vi "Atto DRY Interface upload Temperature Calibration Curve.vi"(8 "error in (no error)":errorcluster, 10 "Path":string, 11 "UserCurveNumber":u8) -> (0 "error out":errorcluster, 2 "Path out":string, 3 "function return":i32)   [LabVIEW 2016, in "attoDRYLib.lvlib"]
doc: "int32_t __cdecl AttoDRY_Interface_uploadTemperatureCalibrationCurve(\n uint8_t UserCurveNumber, char Path[]);"
uses:
  <userlib>/attoDRYLib/attoDRYLib.lvlib
  <userlib>/attoDRYLib/attoDRYLib.dll
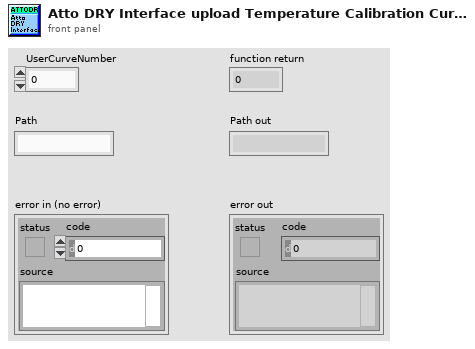
[diagram p1: front panel]
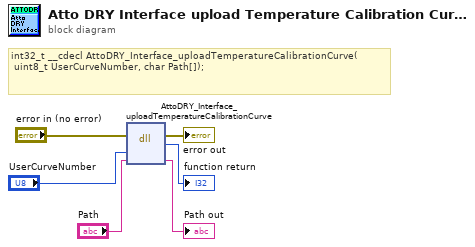
[diagram p0: block diagram]
diagram:
  # "int32_t __cdecl AttoDRY_Interface_uploadTemperatureCalibrationCurve(\n\tuint8_t UserCurveNumber, char Path[]);"
  n1 = dll-call lib="C:/Program Files (x86)/National Instruments/LabVIEW 2016/user.lib/attoDRYLib/attoDRYLib.*" fn="AttoDRY_Interface_uploadTemperatureCalibrationCurve"(error in="error in (no error)", "UserCurveNumber"="UserCurveNumber", "Path"="Path") -> (error out=→"error out":errorcluster, →"function return":i32, "Path"=→"Path out":string)  [unwired: 3 in, 1 out]
